vi "handler_test.vi"(7 "Handler action":enum16{"configure"}(ring)) -> (2 "String":string)   [LabVIEW 2011]
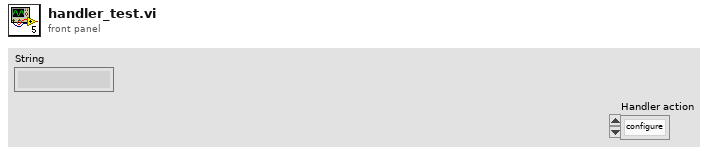
[diagram p1: front panel]
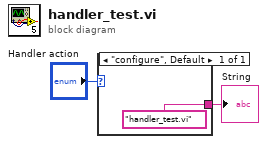
[diagram p0: block diagram]
diagram:
  n1 = case shown="\"configure\", Default" "Handler action" {
    tunnel: ["handler_test.vi"] -> w1
    frame "configure", Default {
    }
  }
  "String" <- w1
